vi "Return var.vi"(8 "error in (no error)":errorcluster, 11 "connection ID":refnum<k5>) -> (0 "error out":errorcluster, 2 "output cluster":cluster{"Name":string, "Data":variant}, 3 "connection ID out":refnum<k5>)   [LabVIEW 2010, in "Matlab API.lvlib"]
uses:
  Matlab API.lvlib
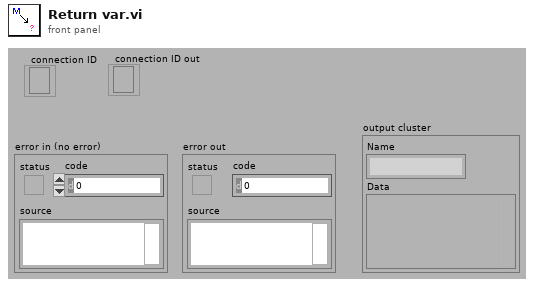
[diagram p1: front panel]
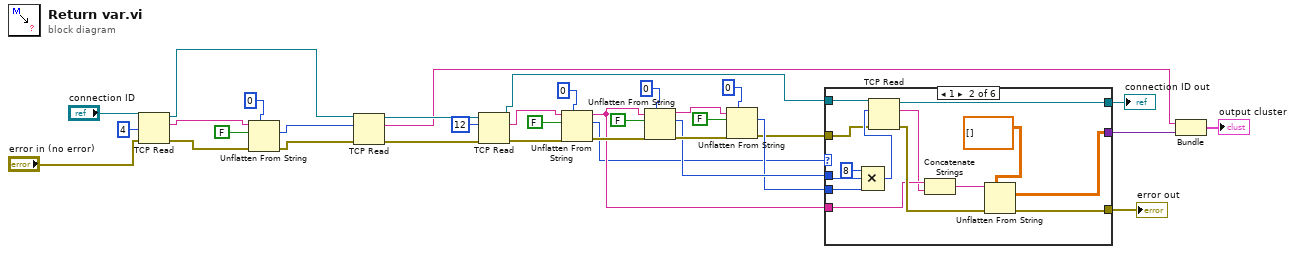
[diagram p0: block diagram]
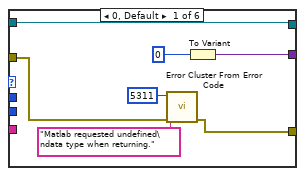
[diagram p2: hidden frame]
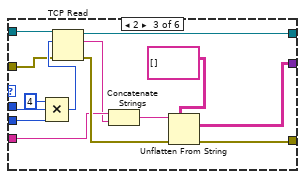
[diagram p3: hidden frame]
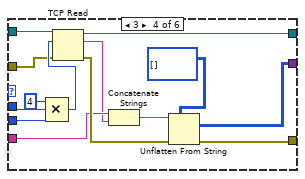
[diagram p4: hidden frame]
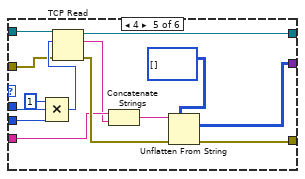
[diagram p5: hidden frame]
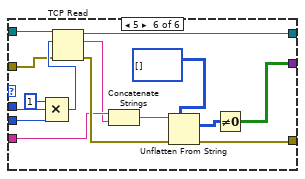
[diagram p6: hidden frame]
diagram:
  n1 = TCP Read(connection ID="connection ID", bytes to read=4, error in (no error)="error in (no error)") -> (connection ID out=w27:refnum<k5>, data out=w30:string, error out=w29:errorcluster)  [unwired: 2 out]
  n2 = Unflatten From String(type=0, binary string=w30, data includes array or string size? (T)=FALSE, error in (no error)=w29) -> (value=w26:i32, error out=w28:errorcluster)  [unwired: 2 out]
  n3 = TCP Read(connection ID=w27, bytes to read=w26, error in (no error)=w28) -> (connection ID out=w24:refnum<k5>, data out=w3:string, error out=w25:errorcluster)  [unwired: 2 out]
  n4 = TCP Read(connection ID=w24, bytes to read=12, error in (no error)=w25) -> (connection ID out=w11:refnum<k5>, data out=w20:string, error out=w19:errorcluster)  [unwired: 1 in, 1 out]
  n5 = Unflatten From String(type=0, binary string=w20, data includes array or string size? (T)=FALSE, error in (no error)=w19) -> (rest of the binary string=w7:string, value=w5:i32, error out=w16:errorcluster)  [unwired: 1 out]
  n6 = Unflatten From String(type=0, binary string=w7, data includes array or string size? (T)=FALSE, error in (no error)=w16) -> (rest of the binary string=w14:string, value=w10:i32, error out=w15:errorcluster)  [unwired: 1 out]
  n7 = Unflatten From String(type=0, binary string=w14, data includes array or string size? (T)=FALSE, error in (no error)=w15) -> (value=w9:i32, error out=w8:errorcluster)  [unwired: 2 out]
  n8 = case shown="1" w5 {
    tunnel: [w41 w56 w70 w84 w98 w113] -> w2
    tunnel: [w39 w54 w68 w82 w96 w99] -> w4
    tunnel: w11 -> [w38 w50 w64 w78 w92 w108]
    tunnel: w10 -> [_ w52 w66 w80 w94 w110]
    tunnel: w9 -> [_ w53 w67 w81 w95 w111]
    tunnel: w8 -> [w37 w48 w62 w76 w90 w106]
    tunnel: w7 -> [_ w45 w59 w73 w87 w103]
    tunnel: [w38 w43 w57 w71 w85 w101] -> w6
    frame 0, Default {
      n9 = call <vilib>:"Error Cluster From Error Code.vi"("error in (no error)"=w37, "error message (\"\")"="Matlab requested undefined\ndata type when returning." ("error message (\"\")"), "error code (0)"=5311) -> ("error out"=w41:errorcluster)  [unwired: 1 in, 5 out]
      n10 = To Variant(anything=0) -> (Variant=w39:variant)
    }
    frame 1 {
      n11 = Compound Arithmetic op=MULTIPLY(8 ("value"), w52, w53) -> (w49:i32)
      n12 = TCP Read(connection ID=w50, bytes to read=w49, error in (no error)=w48) -> (connection ID out=w43:refnum<k5>, data out=w44:string, error out=w47:errorcluster)  [unwired: 1 in, 1 out]
      n13 = Concatenate Strings(w45, w44) -> (w46:string)
      n14 = Unflatten From String(type=dbl[][] [], binary string=w46, error in (no error)=w47) -> (value=w54:dbl[][], error out=w56:errorcluster)  [unwired: 3 out]
    }
    frame 2 {
      n15 = Compound Arithmetic op=MULTIPLY(4 ("value"), w66, w67) -> (w63:i32)
      n16 = TCP Read(connection ID=w64, bytes to read=w63, error in (no error)=w62) -> (connection ID out=w57:refnum<k5>, data out=w58:string, error out=w61:errorcluster)  [unwired: 1 in, 1 out]
      n17 = Concatenate Strings(w59, w58) -> (w60:string)
      n18 = Unflatten From String(type=string[][] [], binary string=w60, error in (no error)=w61) -> (value=w68:string[][], error out=w70:errorcluster)  [unwired: 3 out]
    }
    frame 3 {
      n19 = Compound Arithmetic op=MULTIPLY(4 ("value"), w80, w81) -> (w77:i32)
      n20 = TCP Read(connection ID=w78, bytes to read=w77, error in (no error)=w76) -> (connection ID out=w71:refnum<k5>, data out=w72:string, error out=w75:errorcluster)  [unwired: 1 in, 1 out]
      n21 = Concatenate Strings(w73, w72) -> (w74:string)
      n22 = Unflatten From String(type=i32[][] [], binary string=w74, error in (no error)=w75) -> (value=w82:i32[][], error out=w84:errorcluster)  [unwired: 3 out]
    }
    frame 4 {
      n23 = Compound Arithmetic op=MULTIPLY(1 ("value"), w94, w95) -> (w91:i32)
      n24 = TCP Read(connection ID=w92, bytes to read=w91, error in (no error)=w90) -> (connection ID out=w85:refnum<k5>, data out=w86:string, error out=w89:errorcluster)  [unwired: 1 in, 1 out]
      n25 = Concatenate Strings(w87, w86) -> (w88:string)
      n26 = Unflatten From String(type=u8[][] [], binary string=w88, error in (no error)=w89) -> (value=w96:u8[][], error out=w98:errorcluster)  [unwired: 3 out]
    }
    frame 5 {
      n27 = Compound Arithmetic op=MULTIPLY(1 ("value"), w110, w111) -> (w107:i32)
      n28 = TCP Read(connection ID=w108, bytes to read=w107, error in (no error)=w106) -> (connection ID out=w101:refnum<k5>, data out=w102:string, error out=w105:errorcluster)  [unwired: 1 in, 1 out]
      n29 = Concatenate Strings(w103, w102) -> (w104:string)
      n30 = Unflatten From String(type=u8[][] [], binary string=w104, error in (no error)=w105) -> (value=w100:u8[][], error out=w113:errorcluster)  [unwired: 3 out]
      n31 = Not Equal To 0?(x=w100) -> (x != 0?=w99:bool[][])
    }
  }
  "error out" <- w2
  "connection ID out" <- w6
  n32 = Bundle("data out"=w3, "Variant"=w4) -> (→"output cluster":cluster{"data out":string, "Variant":variant})  [unwired: 1 out]
